vi "SuperNS_GetAttributes.vi"(0 "reference in":refnum<class "SuperNS.lvclass">, 1 "OnlyGetDvrReference(False)":bool, 5 "error in":errorcluster) -> (14 "reference out":refnum<class "SuperNS.lvclass">, 15 "Data":T1 {"Flush Wait Condition" items=["All Elements Read From Stream", "All Elements Available for Reading"]; "Element Allocation Mode" items=["allocate as needed", "pre-allocate"]}, 17 "DataRef":refnum<data-value>, 19 "error out":errorcluster)   [LabVIEW 2020, in "SuperNS.lvclass"]
doc: "Copyright © 2008 - 2024 VI Technologies B.V. \nALL RIGHTS RESERVED"
uses:
  SuperNS.lvclass
  protected/ObjectAttributes.ctl
  <vilib>/dex/Stream Element Allocation Mode.ctl
  <vilib>/dex/Flush And Wait Empty Condition.ctl
  StreamDataType.ctl
  SuperNS.lvclass/SuperNS.ctl
panel:
  # "Copyright (c) 2024, VI Technologies B.V.\nAll rights reserved.\n\nRedistribution and use in source and binary forms, with or without modification, are permitted provided that \nthe following conditions are met:\n\n * Redistributions of source code must retain the above copyright notice, this list of conditions and the \nfollowing disclaimer.\n * Redistributions in binary form must reproduce the above copyright notice, this list of conditions and the \nfollowing disclaimer in the documentation and/or other materials provided with the distribution.\n * Neither the name of VI Technologies B.V. nor the names of its contributors may be used to endorse or \npromote products derived from this software without specific prior written permission.\n\nTHIS SOFTWARE IS PROVIDED BY THE COPYRIGHT HOLDERS AND CONTRIBUTORS \"AS IS\" AND ANY EXPRESS OR \nIMPLIED WARRANTIES, INCLUDING, BUT NOT LIMITED TO, THE IMPLIED WARRANTIES OF MERCHANTABILITY \nAND FITNESS FOR A PARTICULAR PURPOSE ARE DISCLAIMED. IN NO EVENT SHALL THE COPYRIGHT OWNER OR \nCONTRIBUTORS BE LIABLE FOR ANY DIRECT, INDIRECT, INCIDENTAL, SPECIAL, EXEMPLARY, OR CONSEQUENTIAL \nDAMAGES (INCLUDING, BUT NOT LIMITED TO, PROCUREMENT OF SUBSTITUTE GOODS OR SERVICES; LOSS OF \nUSE, DATA, OR PROFITS; OR BUSINESS INTERRUPTION) HOWEVER CAUSED AND ON ANY THEORY OF LIABILITY, \nWHETHER IN CONTRACT, STRICT LIABILITY, OR TORT (INCLUDING NEGLIGENCE OR OTHERWISE) ARISING IN ANY \nWAY OUT OF THE USE OF THIS SOFTWARE, EVEN IF ADVISED OF THE POSSIBILITY OF SUCH DAMAGE.\n\nFor more information, please visit https://www.vi-tech.nl or contact us at info@vi-tech.nl"
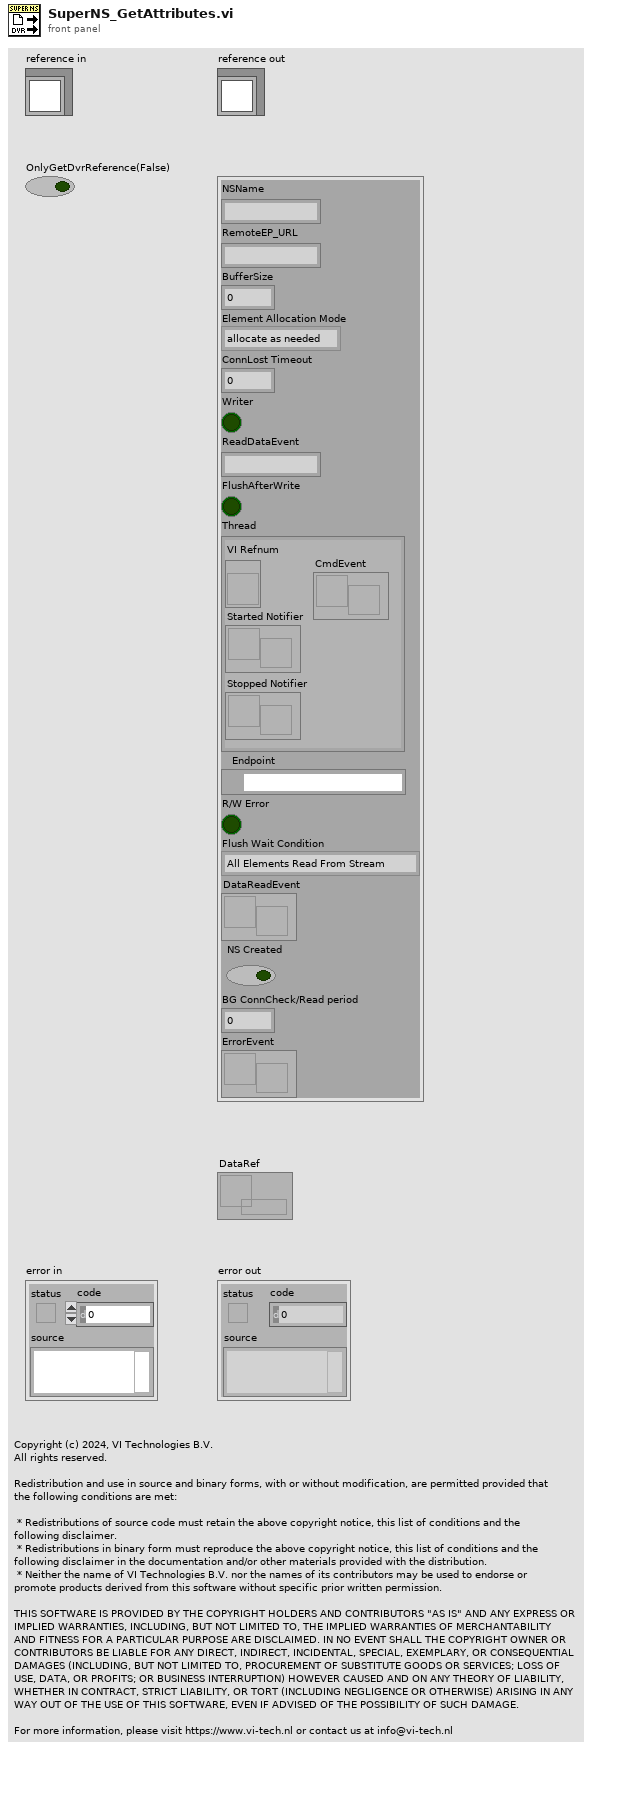
[diagram p1: front panel]
types:
  T1 = typedef "SuperNS.lvclass/ObjectAttributes.ctl" = cluster{"NSName":string, "RemoteEP_URL":string, "BufferSize":i32, "Element Allocation Mode":T2, "ConnLost Timeout":i32, "Writer":bool, "ReadDataEvent":string, "FlushAfterWrite":bool, "Thread":cluster{"VI Refnum":refnum<vi>, "Started Notifier":refnum<notifier>, "Stopped Notifier":refnum<notifier>, "CmdEvent":refnum<user-event>}, "Endpoint":refnum<k21>, "R/W Error":bool, "Flush Wait Condition":T3, "DataReadEvent":refnum<user-event>, "NS Created":bool, "BG ConnCheck/Read period":i32, "ErrorEvent":refnum<user-event>}
  T2 = typedef "Stream Element Allocation Mode.ctl" = u32
  T3 = typedef "Flush And Wait Empty Condition.ctl" = u8
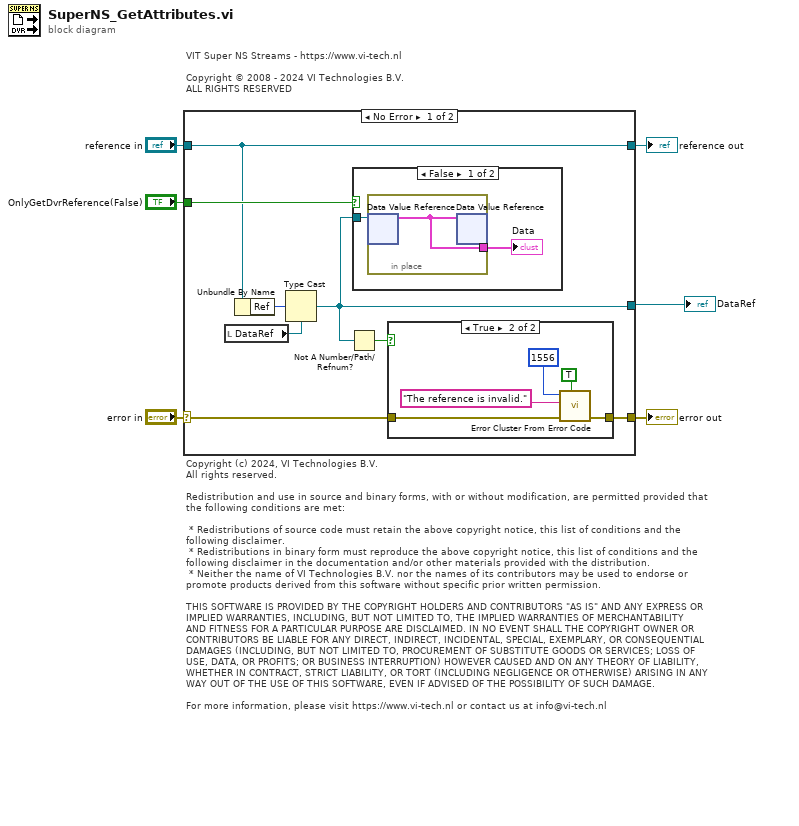
[diagram p0: block diagram]
diagram:
  # "VIT Super NS Streams - https://www.vi-tech.nl\n\nCopyright © 2008 - 2024 VI Technologies B.V. \nALL RIGHTS RESERVED"
  # "Copyright (c) 2024, VI Technologies B.V.\nAll rights reserved.\n\nRedistribution and use in source and binary forms, with or without modification, are permitted provided that \nthe following conditions are met:\n\n * Redistributions of source code must retain the above copyright notice, this list of conditions and the \nfollowing disclaimer.\n * Redistributions in binary form must reproduce the above copyright notice, this list of conditions and the \nfollowing disclaimer in the documentation and/or other materials provided with the distribution.\n * Neither the name of VI Technologies B.V. nor the names of its contributors may be used to endorse or \npromote products derived from this software without specific prior written permission.\n\nTHIS SOFTWARE IS PROVIDED BY THE COPYRIGHT HOLDERS AND CONTRIBUTORS \"AS IS\" AND ANY EXPRESS OR \nIMPLIED WARRANTIES, INCLUDING, BUT NOT LIMITED TO, THE IMPLIED WARRANTIES OF MERCHANTABILITY \nAND FITNESS FOR A PARTICULAR PURPOSE ARE DISCLAIMED. IN NO EVENT SHALL THE COPYRIGHT OWNER OR \nCONTRIBUTORS BE LIABLE FOR ANY DIRECT, INDIRECT, INCIDENTAL, SPECIAL, EXEMPLARY, OR CONSEQUENTIAL \nDAMAGES (INCLUDING, BUT NOT LIMITED TO, PROCUREMENT OF SUBSTITUTE GOODS OR SERVICES; LOSS OF \nUSE, DATA, OR PROFITS; OR BUSINESS INTERRUPTION) HOWEVER CAUSED AND ON ANY THEORY OF LIABILITY, \nWHETHER IN CONTRACT, STRICT LIABILITY, OR TORT (INCLUDING NEGLIGENCE OR OTHERWISE) ARISING IN ANY \nWAY OUT OF THE USE OF THIS SOFTWARE, EVEN IF ADVISED OF THE POSSIBILITY OF SUCH DAMAGE.\n\nFor more information, please visit https://www.vi-tech.nl or contact us at info@vi-tech.nl"
  n1 = case shown="No Error" "error in" {
    selector: "error in" -> [w14 w25]
    tunnel: [w13 w25] -> w5
    tunnel: [w8 w24] -> w3
    tunnel: "reference in" -> [w8 w24]
    tunnel: [w10 _] -> w1
    tunnel: "OnlyGetDvrReference(False)" -> [w11 _]
    frame No Error {
      n2 = local read "DataRef"() -> (w7:refnum<data-value>)
      n3 = Unbundle By Name(w8) -> ("Ref"=w12:u32)
      n4 = Type Cast(type=w7, x=w12) -> (*(type *) &x=w10:refnum<data-value>)
      n5 = Not A Number/Path/Refnum?(number/path/refnum=w10) -> (NaN/Path/Refnum?=w9:bool)
      n6 = case shown="False" w11 {
        tunnel: w10 -> [w22 _]
        frame False {
          n7 = in-place {
            in-place-border: [w23] -> w21
            n8 = in-place-dvr #1(w22) -> (w23:T1)  [unwired: 1 out]
            n9 = in-place-dvr #1(w23) -> ()  [unwired: 2 out]
          }
          "Data" <- w21
        }
        frame True {
        }
      }
      n10 = case shown="True" w9 {
        tunnel: w14 -> [w15 w20]
        tunnel: [w15 w19] -> w13
        frame False {
        }
        frame True {
          n11 = call <vilib>:"Error Cluster From Error Code.vi"("show call chain? (False)"=TRUE, "error in (no error)"=w20, "error message (\"\")"="The reference is invalid." ("source"), "error code (0)"=1556 ("code")) -> ("error out"=w19:errorcluster)  [unwired: 5 in]
        }
      }
    }
    frame Error {
    }
  }
  "error out" <- w5
  "reference out" <- w3
  "DataRef" <- w1
